vi "Regroup Command Line Arguments.vi"(10 "CLI Arguments":string[](array[string])) -> (1 "Remaining Args":string[](array[string]), 2 "Options":variant)   [LabVIEW 2014]
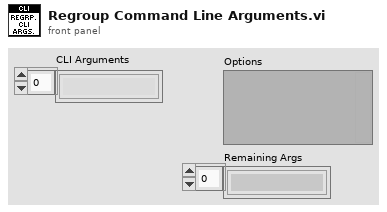
[diagram p1: front panel]
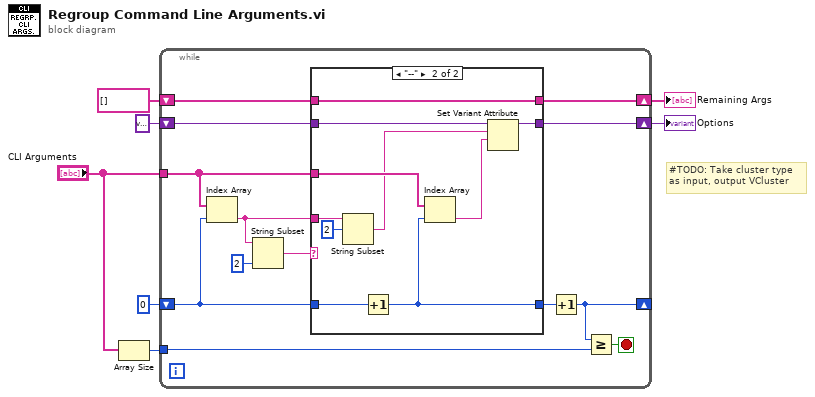
[diagram p0: block diagram]
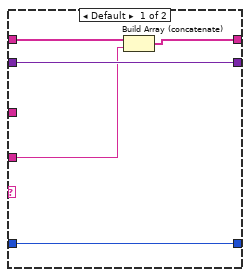
[diagram p2: hidden frame]
diagram:
  # "#TODO: Take cluster type\nas input, output VCluster"
  n1 = Array Size(array="CLI Arguments") -> (size(s)=w4:i32)
  n2 = while {
    shift-right: [w12] -> _
    shift-left: 0 -> [w16]
    tunnel: "CLI Arguments" -> [w17]
    shift-right: [w14] -> w2
    shift-left: variant -> [w15]
    tunnel: w4 -> [w11]
    shift-right: [w8] -> w1
    shift-left: string[] [] -> [w9]
    stop <- w10 stop-if-true
    n3 = Index Array(array=w17, index=w16) -> (element=w18:string)
    n4 = String Subset(string=w18, length (rest)=2 ("length (rest)")) -> (substring=w19:string)  [unwired: 1 in]
    n5 = case shown="\"--\"" w19 {
      tunnel: w18 -> [w22 w35]
      tunnel: w17 -> [_ w33]
      tunnel: w16 -> [w25 w32]
      tunnel: w15 -> [w24 w31]
      tunnel: [w24 w28] -> w14
      tunnel: [w25 w27] -> w13
      tunnel: w9 -> [w23 w26]
      tunnel: [w21 w26] -> w8
      frame Default {
        n6 = Build Array (concatenate)(w23, w22) -> (w21:string[])
      }
      frame "--" {
        n7 = String Subset(string=w35, offset (0)=2) -> (substring=w30:string)  [unwired: 1 in]
        n8 = Increment(x=w32) -> (x+1=w27:i32)
        n9 = Index Array(array=w33, index=w27) -> (element=w29:string)
        n10 = Set Variant Attribute(Variant=w31, name=w30, value=w29) -> (Variant out=w28:variant)  [unwired: 1 in, 2 out]
      }
    }
    n11 = Increment(x=w13) -> (x+1=w12:i32)
    n12 = Greater Or Equal?(x=w12, y=w11) -> (x >= y?=w10:bool)
  }
  "Options" <- w2
  "Remaining Args" <- w1
